vi "CRYString all white space.vi"(11 "String":string) -> (3 "Nothing but white space?":bool)   [LabVIEW 2013]
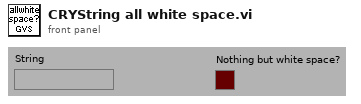
[diagram p1: front panel]
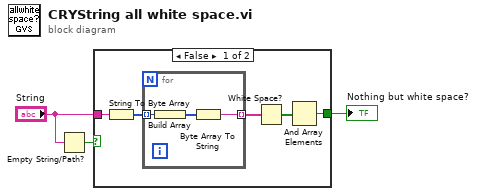
[diagram p0: block diagram]
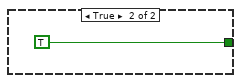
[diagram p2: hidden frame]
diagram:
  n1 = Empty String/Path?(string/path="String") -> (empty?=w1:bool)
  n2 = case shown="False" w1 {
    tunnel: "String" -> [w8 _]
    tunnel: [w4 TRUE] -> w3
    frame False {
      n3 = String To Byte Array(string=w8) -> (unsigned byte array=w7:u8[])
      n4 = for {
        tunnel: w7 -> [w11] mode=indexing
        tunnel: [w9] -> w6 mode=indexing
        n5 = Build Array(w11) -> (w10:u8[])
        n6 = Byte Array To String(unsigned byte array=w10) -> (string=w9:string)
      }
      n7 = White Space?(1:w6) -> (0:w5:bool[])
      n8 = And Array Elements(Boolean array=w5) -> (logical AND=w4:bool)
    }
    frame True {
    }
  }
  "Nothing but white space?" <- w3
